vi "check_start_conditions_flexRIO.vi"(4 "FIFO overflow?":bool, 6 "stop at FIFO overflow?":bool, 9 "already acquiring?":bool, 10 "in triggered mode?":bool, 11 "acquire":bool) -> (2 "acquire?":bool)   [LabVIEW 2010]
uses:
  <vilib>/eio/EIONode/EIONode.xnode
  <vilib>/rvi/eio/nirviEIOImplementation/nirviEIOImplementation.xnode
  <vilib>/rvi/eio/common/nirviEmuClasses.ctl
  <vilib>/rvi/eio/common/nirviEmuTemplateMethod_noerrors.vi
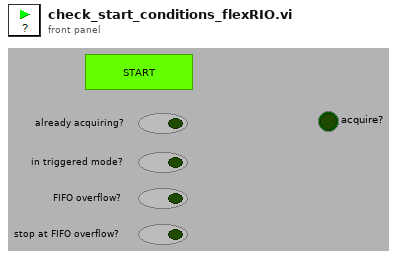
[diagram p1: front panel]
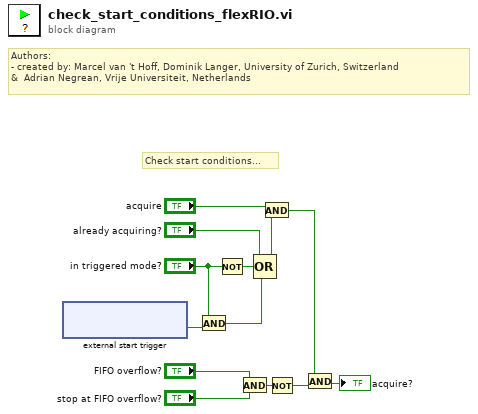
[diagram p0: block diagram]
diagram:
  # "Authors: \n- created by: Marcel van 't Hoff, Dominik Langer, University of Zurich, Switzerland\n&  Adrian Negrean, Vrije Universiteit, Netherlands"
  # "Check start conditions..."
  n1 = xnode "external start trigger"() -> ("IO Module\\DI 0"=w1:bool)  [unwired: 1 in, 1 out]
  n2 = And(x="in triggered mode?", y=w1) -> (x .and. y?=w9:bool)
  n3 = Not(x="in triggered mode?") -> (.not. x?=w11:bool)
  n4 = And(x="FIFO overflow?", y="stop at FIFO overflow?") -> (x .and. y?=w6:bool)
  n5 = Compound Arithmetic op=OR("already acquiring?", w11, w9) -> (w13:bool)
  n6 = And(x="acquire", y=w13) -> (x .and. y?=w4:bool)
  n7 = Not(x=w6) -> (.not. x?=w5:bool)
  n8 = And(x=w4, y=w5) -> (x .and. y?=→"acquire?":bool)
